vi "CDMA_RxDespread.vi"(6 "sampleRate":dbl, 7 "ch_code_rx":dbl, 8 "error in (no error)":errorcluster caption="错误输入（无错误）", 9 "ch_sf_rx":dbl, 10 "rx_data1":cdb[](array[numeric]), 11 "Path In":path) -> (0 "error out":errorcluster caption="错误输出", 2 "pichData":cdb[](array[numeric]), 3 "Path Out":path)   [LabVIEW 2015]
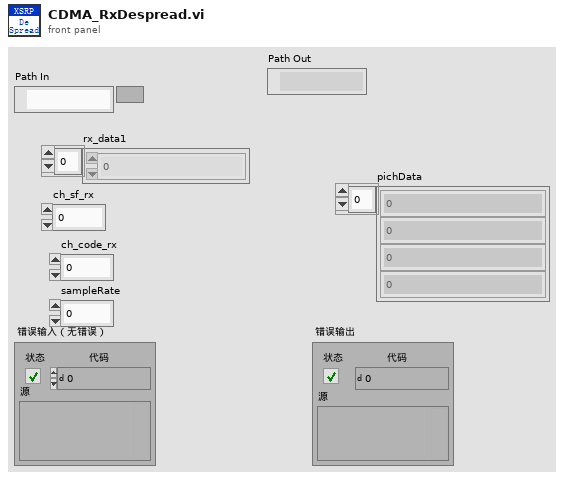
[diagram p1: front panel]
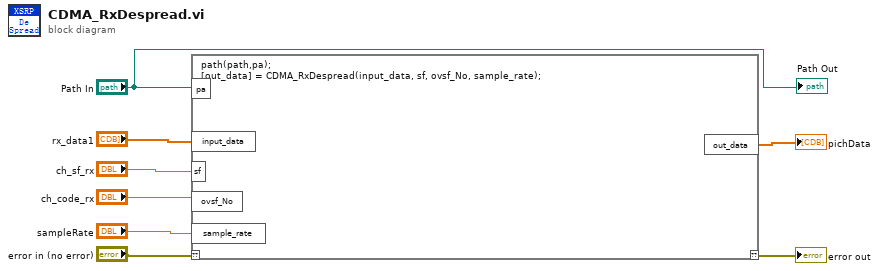
[diagram p0: block diagram]
diagram:
  n1 = script code="path(path,pa);\n[out_data] = CDMA_RxDespread(input_data, sf, ovsf_No, sample_rate);"("??"="error in (no error)", "pa"="Path In", "input_data"="rx_data1", "sf"="ch_sf_rx", "ovsf_No"="ch_code_rx", "sample_rate"="sampleRate") -> ("??"=→"error out":errorcluster, "out_data"=→"pichData":cdb[])
  "Path Out" <- "Path In"
